vi "NI VeriStand - Get Custom Device Channel Scale Units.vi"(8 "error in (no error)":errorcluster, 11 "Device Ref in":T1 format="%.0x") -> (0 "error out":errorcluster, 2 "ScaleUnits":string, 3 "Device Ref out":T1 format="%.0x")   [LabVIEW 2020, in "Custom Device Offline API.lvlib"]
uses:
  <vilib>/NI VeriStand/Custom Device Offline API/Custom Device Offline API.lvlib
  <vilib>/NI VeriStand/Custom Device API/Custom Device Item Ref.ctl
  NationalInstruments.VeriStand.SystemDefinitionAPI
  <vilib>/NI VeriStand/Custom Device API/Custom Device API.lvlib
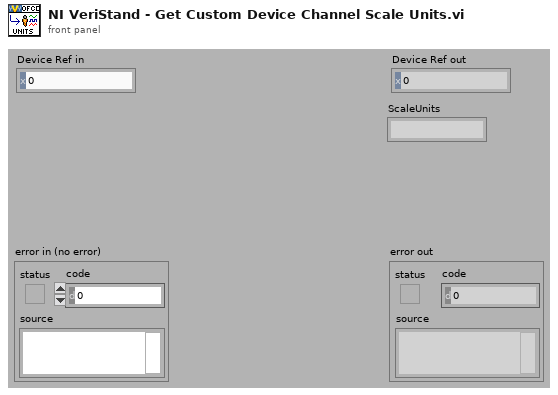
[diagram p1: front panel]
types:
  T1 = typedef "Custom Device API.lvlib/Custom Device Item Ref.ctl" = u64
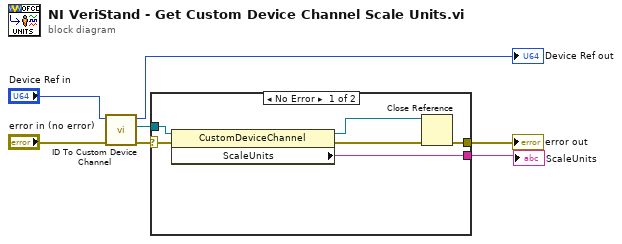
[diagram p0: block diagram]
diagram:
  n1 = call <vilib>:"ID To Custom Device Channel.vi"("error in (no error)"="error in (no error)", "ID in"="Device Ref in") -> ("error out"=w5:errorcluster, "Channel"=w2:refnum<k24>, "ID out"=→"Device Ref out":u64)  [unwired: 7 in]
  n2 = case shown="No Error" w5 {
    selector: w5 -> [w11 w14]
    tunnel: [w13 w14] -> w7
    tunnel: w2 -> [w12 _]
    tunnel: [w8 _] -> w1
    frame No Error {
      n3 = property class="CustomDeviceChannel"(reference=w12, error in=w11) -> (reference out=w9:refnum<k24>, error out=w10:errorcluster, "ScaleUnits"=w8:string)
      n4 = Close Reference(reference=w9, error in (no error)=w10) -> (error out=w13:errorcluster)
    }
    frame Error {
    }
  }
  "error out" <- w7
  "ScaleUnits" <- w1
